vi "Motor Output Global.vi"() -> ()   [LabVIEW 2009]
panel:
  in  "Lidar Output Command":fxp<+/-,20,5>
  in  "Steering Output Command":fxp<+/-,20,5>
  in  "Drive Output Command":fxp<+/-,20,5>
  in  "Lidar Output Voltage":fxp<+/-,20,5>
  in  "Steering Output Voltage":fxp<+/-,20,5>
  in  "Drive Output Voltage":fxp<+/-,20,5>
  out "Drive Reverse":bool
  out "Lidar Enable":bool
  out "Steering Enable":bool
  out "Drive Enable":bool
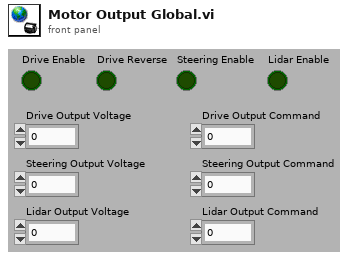
[diagram p1: front panel]
diagram:
